vi "Setup.vi"(8 "Error In":errorcluster, 9 "Password":string, 10 "Username":string, 11 "Address":string) -> (0 "Error Out":errorcluster, 2 "Temporary Directory":string, 3 "SFTP":refnum<class "SFTP.lvclass">)   [LabVIEW 2018, in "Tests.lvlib" / "SFTP Directory.lvlib"]
uses:
  SFTP Directory.lvlib
  src/Toolkit/SFTP/SFTP.lvclass
  src/Toolkit/Session/Support/Password Authentication.vi
  src/Toolkit/SSH/SSH.lvclass
  src/Toolkit/Session/Session.lvclass
  Tests.lvlib
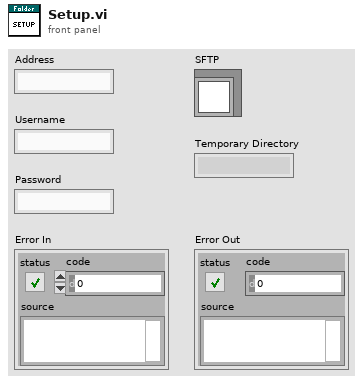
[diagram p1: front panel]
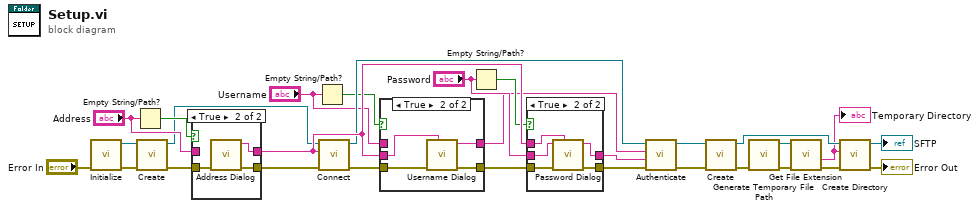
[diagram p0: block diagram]
diagram:
  n1 = call "Initialize.vi"("Error In"="Error In") -> ("Error Out"=w10:errorcluster, "SSH"=w11:refnum<class "SSH.lvclass">)  [unwired: 9 in]
  n2 = Empty String/Path?(string/path="Address") -> (empty?=w14:bool)
  n3 = call "Create.vi"("Error In"=w10, "SSH"=w11) -> ("Error Out"=w16:errorcluster, "Sesssion"=w13:refnum<class "Session.lvclass">)  [unwired: 8 in]
  n4 = case shown="True" w14 {
    tunnel: w16 -> [w30 w34]
    tunnel: [w30 w33] -> w17
    tunnel: [w31 w32] -> w29
    tunnel: "Address" -> [w31 _]
    frame False {
    }
    frame True {
      n5 = call "Address Dialog.vi"("Error In"=w34) -> ("Error Out"=w33:errorcluster, "Address Out"=w32:string)  [unwired: 9 in]
    }
  }
  n6 = Empty String/Path?(string/path="Username") -> (empty?=w22:bool)
  n7 = call "Connect.vi"("Error In"=w17, "Address"=w29, "Session In"=w13) -> ("Error Out"=w25:errorcluster, "Sesssion Out"=w28:refnum<class "Session.lvclass">)  [unwired: 7 in]
  n8 = case shown="True" w22 {
    tunnel: w25 -> [w36 w40]
    tunnel: [w35 w39] -> w9
    tunnel: [w36 w38] -> w18
    tunnel: "Username" -> [w35 _]
    tunnel: w29 -> [_ w37]
    frame False {
    }
    frame True {
      n9 = call "Username Dialog.vi"("Address"=w37, "Error In"=w40) -> ("Error Out"=w38:errorcluster, "Username Out"=w39:string)  [unwired: 8 in]
    }
  }
  n10 = Empty String/Path?(string/path="Password") -> (empty?=w24:bool)
  n11 = case shown="True" w24 {
    tunnel: "Password" -> [w42 w47]
    tunnel: w18 -> [w41 w46]
    tunnel: [w41 w45] -> w19
    tunnel: [w42 w44] -> w20
    tunnel: w29 -> [_ w43]
    frame False {
    }
    frame True {
      n12 = call "Password Dialog.vi"("Address"=w43, "Error In"=w46, "Password In"=w47) -> ("Error Out"=w45:errorcluster, "Password Out"=w44:string)  [unwired: 7 in]
    }
  }
  n13 = call-poly "Authenticate.vi"("Error In"=w19, "Password"=w20, "Username"=w9, "Session In"=w28) -> ("Error Out"=w26:errorcluster, "Sesssion Out"=w27:refnum<class "Session.lvclass">)  [unwired: 6 in]
  n14 = call "Create.vi"("Error In"=w26, "Session"=w27) -> ("Error Out"=w5:errorcluster, "SFTP"=w2:refnum<class "SFTP.lvclass">)  [unwired: 8 in]
  n15 = call <vilib>:"Generate Temporary File Path.vi"("error in (no error)"=w5) -> ("error out"=w7:errorcluster, "Unique Temporary File Path"=w8:path)  [unwired: 9 in]
  n16 = call <vilib>:"Get File Extension.vi"("error in (no error)"=w7, "file"=w8) -> ("error out"=w6:errorcluster, "filename without extension"=w1:string)  [unwired: 5 in, 3 out]
  "Temporary Directory" <- w1
  n17 = call "Create Directory.vi"("Error In"=w6, "Remote Path"=w1, "SFTP In"=w2) -> ("Error Out"=→"Error Out":errorcluster, "SFTP Out"=→"SFTP":refnum<class "SFTP.lvclass">)  [unwired: 7 in]
